vi "post semaphores.vi"(8 "error in (no error)":errorcluster, 11 "semaphores in":T1[](array[typedef])) -> (0 "error out":errorcluster, 3 "semaphores out":T1[](array[typedef]))   [LabVIEW 2013, in "Shared Memory runtime.lvclass"]
uses:
  Shared Memory runtime.lvclass
  controls/semaphore data.ctl
  <vilib>/NI/Pthreads for LabVIEW on Linux RT/Classes/Semaphore/Controls/reference.ctl
  <vilib>/NI/Pthreads for LabVIEW on Linux RT/Classes/Semaphore/Semaphore.lvclass
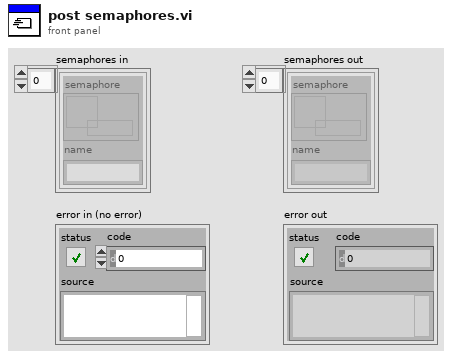
[diagram p1: front panel]
types:
  T1 = typedef "Shared Memory runtime.lvclass/semaphore data.ctl" = cluster{"semaphore":T2, "name":string}
  T2 = typedef "POSIX Threads.lvlib/Semaphore.lvclass/reference.ctl" = refnum<data-value>
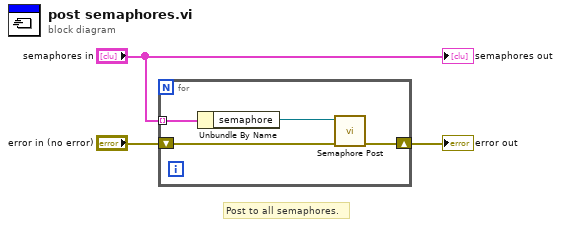
[diagram p0: block diagram]
diagram:
  # "Post to all semaphores."
  n1 = for {
    shift-right: [w6] -> w2
    shift-left: "error in (no error)" -> [w7]
    tunnel: "semaphores in" -> [w5] mode=indexing
    n2 = Unbundle By Name(w5) -> ("semaphore"=w4:T2)
    n3 = call <vilib>:"Semaphore Post.vi"("error in (no error)"=w7, "Semaphore in"=w4) -> ("error out"=w6:errorcluster)  [unwired: 8 in, 1 out]
  }
  "error out" <- w2
  "semaphores out" <- "semaphores in"
